vi "pulse data format.vi"(0 "file path (dialog if empty)":path) -> (1 "time":dbl[](array[numeric]) format="%.8f", 2 "file path read":path=path "/Macintosh HD/Data/Jeremy/RbHg/Rb/s12211.001", 3 "rate of change of field":dbl[](array[numeric]) format="%.3f", 4 "magnetic field":dbl[](array[numeric]) format="%.3f", 5 "signal channel A":dbl[](array[numeric]) format="%.3f", 6 "signal channel B":dbl[](array[numeric]) format="%.3f")   [LabVIEW 2016]
uses:
  <vilib>/Analysis/baseanly.llb/Mean (DBL).vi
  <vilib>/Analysis/2dsp.llb/Derivative x(t).vi
  <vilib>/Analysis/NI_AALBase.lvlib
  <vilib>/Analysis/NI_AALPro.lvlib
panel:
  in  "force int?":bool
  in  "B offset":dbl format="%.2f"
  in  "minutes?":bool
  in  "t shift":dbl=0.4 format="%.2f"
  in  "format":string="%f"
  in  "stop":bool
  in  "tau(s)":dbl=0.1 format="%.2f"
  in  "unfilter?":bool
  in  "tau(s)":dbl=0.03 format="%.2f"
  in  "unfilter?":bool
  in  "inv?":bool
  in  "?":u8(ring)=11 items=["1", "3", "7", "15", "31", "63", "127", "255", "511"]
  in  "fit":u16(ring)=2 items=["none", "linear", "box", "auto"]
  in  "sweep rate":dbl=1.0 format="%.2f"
  in  "inv?":bool
  in  "tolerance":dbl=1.0 format="%.2f"
  in  "col":u8=1 min=1
  in  "edit spikes?":bool
  in  "array conversion":u16(ring) items=["standard tab", " arrbitrary spaces"]
  in  "?":i16
  in  "?":i16
  in  "?":bool
  in  "?":bool
  in  "y axis":u16(ring)=3 items=["time", "rate of change of B", "magnetic field", "signal A", "signal B"]
  in  "x axis":u16(ring)=2 items=["time", "rate of change of B", "magnetic field", "signal A", "signal B"]
  out "plotted data":cluster{dbl[], dbl[]}(graph)
  out "no. of columns":u32=5
  out "no. of rows":u32=32768
  in  "y offset":dbl format="%.3f"
  in  "x offset":dbl format="%.3f"
  in  "y col.":u16=3 min=1 step=1
  in  "x col.":u16=2 min=1 step=1
  in  "signal channel B":u16(ring)=3 items=["spreadsheet column x", "integrate column x with constant", "magnitude of columns x & y", "ignore"]
  in  "y offset":dbl format="%.3f"
  in  "x offset":dbl format="%.3f"
  in  "y col.":u16=3 min=1 step=1
  in  "x col.":u16=2 min=1 step=1
  in  "signal channel A":u16(ring) items=["spreadsheet column x", "integrate column x with constant", "magnitude of columns x & y", "Derivative of x column"]
  in  "pretrigger points":u32=1600 min=1 step=1
  in  "column #":u16=2 min=1 step=1
  in  "magnetic field":u16(ring)=2 items=["spreadsheet column", "integrate using time column", " TLM shunt voltage", "field shift correction", "ignore"]
  in  "calibration constant":dbl=11230.0 format="%.2f"
  in  "column #":u16=4 min=1 step=1
  in  "rate of change of field":u16(ring)=1 items=["spreadsheet column", "renormalize column with calibration", "create from B", "ignore"]
  in  "time interval":dbl=2e-06 min=1e-09 format="%.2p"
  in  "column #":u16=5 min=1 step=1
  in  "time column":u16(ring) items=["spreadsheet column", "create from time interval", "ignore"]
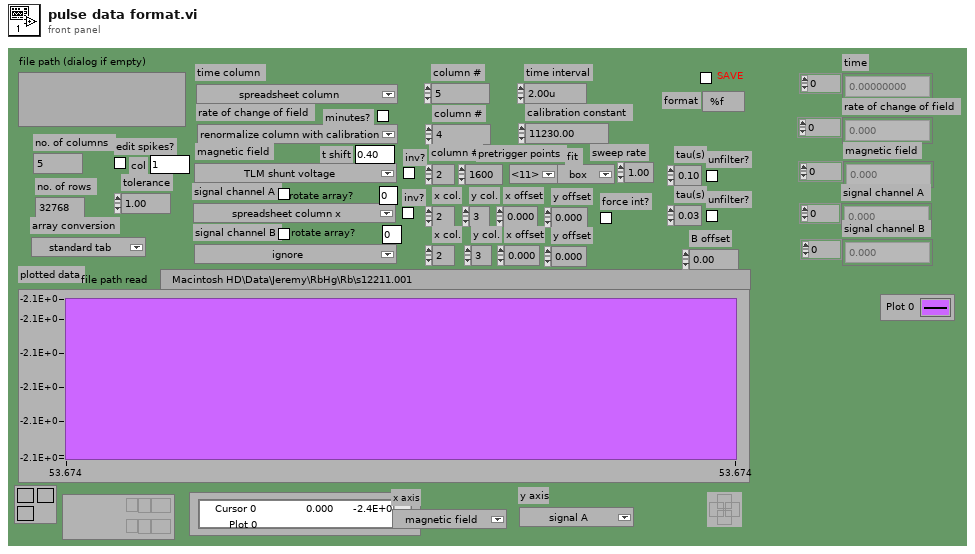
[diagram p1: front panel]
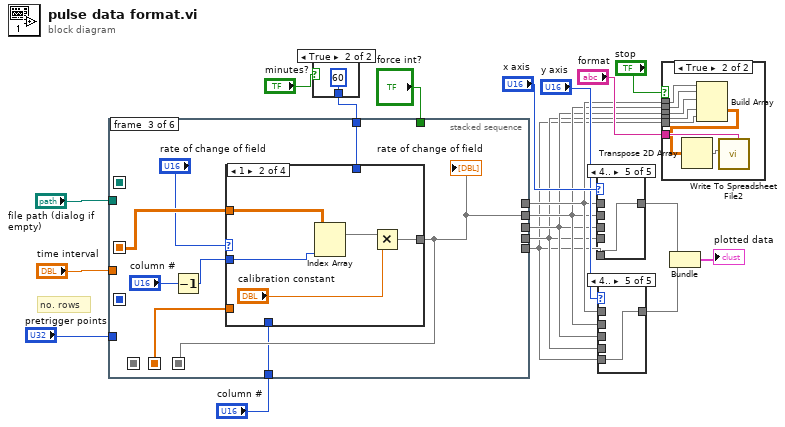
[diagram p0: block diagram]
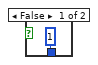
[diagram p2: hidden frame]
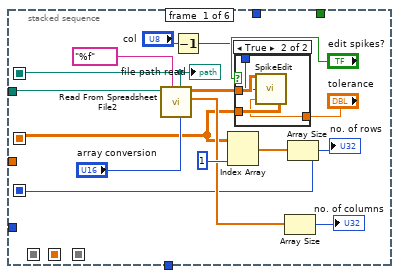
[diagram p12: hidden frame]
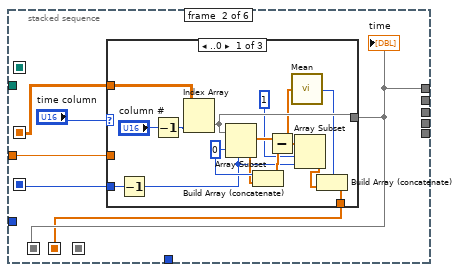
[diagram p14: hidden frame]
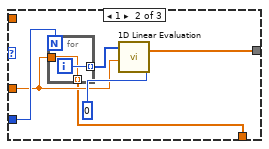
[diagram p15: hidden frame]
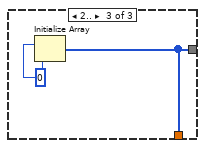
[diagram p16: hidden frame]
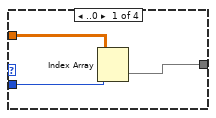
[diagram p17: hidden frame]
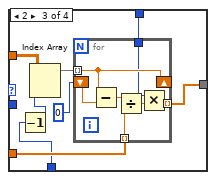
[diagram p18: hidden frame]
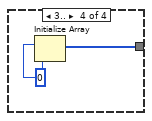
[diagram p19: hidden frame]
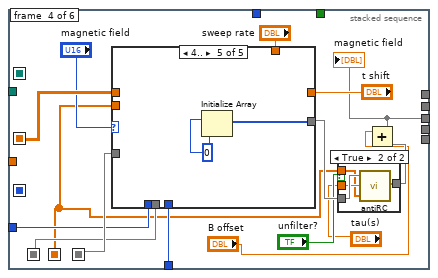
[diagram p20: hidden frame]
diagram:
  # "no. rows"
  n1 = case shown="True" "minutes?" {
    tunnel: [1 60] -> w2
    frame False {
    }
    frame True {
    }
  }
  n2 = stacked-sequence {
    seq-local: [w29 _ _ _ _ _] -> [_ _ _ _ _ _]
    seq-local: [w26 _ _ _ _ _] -> [_ w46 w79 w119 w176 w243]
    seq-local: [w30 _ _ _ _ _] -> [_ w44 _ _ _ _]
    seq-local: [_ w43 _ _ _ _] -> [_ _ _ w117 w162 w232]
    seq-local: [_ _ w75 _ _ _] -> [_ _ _ w118 _ _]
    seq-local: [_ w42 _ _ _ _] -> [_ _ w72 w108 w161 _]
    tunnel: "file path (dialog if empty)" -> [w36 _ _ _ _ _]
    tunnel: "time interval" -> [_ w45 _ _ _ _]
    tunnel: "pretrigger points" -> [_ _ _ w116 w174 w242]
    tunnel: [_ w43 _ _ _ _] -> w9
    tunnel: [_ _ w75 _ _ _] -> w8
    tunnel: [_ _ _ w105 _ _] -> w7
    tunnel: [_ _ _ _ w163 _] -> w6
    tunnel: [_ _ _ _ _ w235] -> w5
    tunnel: "column #" -> [_ _ w74 w109 _ _]
    tunnel: w2 -> [_ _ w73 _ _ _]
    tunnel: "force int?" -> [_ _ _ _ w159 _]
    frame #0 {
      n3 = call "Read From Spreadsheet File2.vi"("array conversion"="array conversion", "format (%.3f)"="%f", "file path (dialog if empty)"=w36) -> ("first row"=w32:sgl[], "all rows"=w27:sgl[][], "new file path (Not A Path if cancelled)"=w29:path)  [unwired: 4 in, 2 out]
      "file path read" <- w29
      n4 = Decrement(x="col") -> (x-1=w23:u8)
      n5 = case shown="True" "edit spikes?" {
        tunnel: w27 -> [w37 w40]
        tunnel: [w37 w41] -> w26
        tunnel: w23 -> [_ w39]
        tunnel: "tolerance" -> [_ w38]
        frame False {
        }
        frame True {
          n6 = call "SpikeEdit.vi"("tolerance"=w38, "column"=w39, "data in"=w40) -> ("data out"=w41:dbl[][])
        }
      }
      n7 = Index Array(array=w26, index (col)=1) -> (element=w33:dbl[])  [unwired: 1 in]
      n8 = Array Size(array=w32) -> (size(s)=→"no. of columns":i32)
      n9 = Array Size(array=w33) -> (size(s)=w30:i32)
      "no. of rows" <- w30
    }
    frame #1 {
      n10 = case shown="..0" "time column" {
        tunnel: [w57 w64 w70] -> w43
        tunnel: w46 -> [w60 _ _]
        tunnel: w45 -> [_ w63 _]
        tunnel: w44 -> [w58 w67 _]
        tunnel: [w48 w62 w70] -> w42
        frame ..0 {
          w56 = 0
          n11 = Decrement(x=w58) -> (x-1=w52:i32)
          n12 = Decrement(x="column #") -> (x-1=w59:u16)
          n13 = Index Array(array=w60, index (col)=w59) -> (element=w57:dbl[])  [unwired: 1 in]
          n14 = Array Subset(array=w57, index=w56, length=w52) -> (w55:dbl[])
          n15 = Build Array (concatenate)(w56, w55) -> (w54:dbl[])
          n16 = Subtract(x=w55, y=w54) -> (x-y=w53:dbl[])
          n17 = call-poly <vilib>:"Mean.vi"("X"=w53) -> ("error"=w50:i32)  [unwired: 1 out]
          n18 = Array Subset(array=w53, index=1, length=w52) -> (w49:dbl[])
          n19 = Build Array (concatenate)(w50, w49) -> (w48:dbl[])
        }
        frame 1 {
          n20 = for {
            N: w67 -> [_]
            tunnel: [w69] -> w66 mode=indexing
            tunnel: w63 -> [w68]
            tunnel: [w68] -> w62 mode=indexing
            i -> [w69]
          }
          n21 = call <vilib>:"1D Linear Evaluation.vi"("offset"=0, "scale"=w63, "X"=w66) -> ("Y[i]=X[i]*a+b"=w64:dbl[])  [unwired: 1 out]
        }
        frame 2.. {
          w71 = 0
          n22 = Initialize Array(w71, w71) -> (w70:i32[])
        }
      }
      "time" <- w43
    }
    frame #2 {
      n23 = Decrement(x="column #") -> (x-1=w76:u16)
      n24 = case shown="1" "rate of change of field" {
        tunnel: [w82 w84 w91 w104] -> w75
        tunnel: w79 -> [w81 w87 w95 _]
        tunnel: w76 -> [w80 w83 _ _]
        tunnel: w72 -> [_ _ w92 _]
        tunnel: w74 -> [_ _ w90 _]
        tunnel: w73 -> [_ _ w88 _]
        frame ..0 {
          n25 = Index Array(array=w81, index (col)=w80) -> (element=w82:dbl[])  [unwired: 1 in]
        }
        frame 1 {
          n26 = Index Array(array=w87, index (col)=w83) -> (element=w85:dbl[])  [unwired: 1 in]
          n27 = Multiply(x=w85, y="calibration constant") -> (x*y=w84:dbl[])
        }
        frame 2 {
          n28 = Decrement(x=w90) -> (x-1=w89:u16)
          n29 = Index Array(array=w95, index (col)=w89) -> (element=w93:dbl[])  [unwired: 1 in]
          n30 = for {
            shift-right: [w102] -> _
            shift-left: 0 -> [w101]
            tunnel: w93 -> [w102] mode=indexing
            tunnel: w92 -> [w99] mode=indexing
            tunnel: [w98] -> w91 mode=indexing
            tunnel: w88 -> [w96]
            n31 = Subtract(x=w102, y=w101) -> (x-y=w100:dbl)
            n32 = Divide(x=w100, y=w99) -> (x/y=w97:dbl)
            n33 = Multiply(x=w96, y=w97) -> (x*y=w98:dbl)
          }
        }
        frame 3.. {
          w103 = 0
          n34 = Initialize Array(w103, w103) -> (w104:i32[])
        }
      }
      "rate of change of field" <- w75
    }
    frame #3 {
      n35 = case shown="4.." "magnetic field" {
        tunnel: [w127 w135 w146 w150 w158] -> w114
        tunnel: w119 -> [w130 _ w149 w154 _]
        tunnel: w116 -> [_ w136 _ _ _]
        tunnel: w118 -> [_ w137 _ _ _]
        tunnel: w108 -> [_ _ _ w151 _]
        tunnel: w117 -> [_ w134 _ _ _]
        tunnel: w109 -> [w126 _ w147 w155 _]
        tunnel: "sweep rate" -> [_ _ w138 _ _]
        tunnel: "t shift" -> [_ _ _ w152 _]
        frame ..0 {
          n36 = Decrement(x=w126) -> (x-1=w129:u16)
          n37 = Index Array(array=w130, index (col)=w129) -> (element=w128:dbl[])  [unwired: 1 in]
          n38 = case shown="True" "inv?" {
            tunnel: w128 -> [w131 w133]
            tunnel: [w131 w132] -> w127
            frame False {
            }
            frame True {
              n39 = Reciprocal(x=w133) -> (1/x=w132:dbl[])
            }
          }
        }
        frame 1 {
          n40 = call "integrator.vi"("pretrigger points"=w136, "time"=w134, "input"=w137) -> ("output"=w135:dbl[])
        }
        frame 2 {
          n41 = Decrement(x=w147) -> (x-1=w148:u16)
          n42 = Index Array(array=w149, index (col)=w148) -> (element=w145:dbl[])  [unwired: 1 in]
          n43 = Increment(x="?") -> (x+1=w142:u8)
          n44 = Scale By Power Of 2(n=w142, x=1) -> (x*2^n=w140:i32)
          n45 = Decrement(x=w140) -> (x-1=w139:i32)
          n46 = call "TLM.vi"("sweep rate (A/min)"=w138, "fit"="fit", "shunt V"=w145, "BOX"=w139) -> ("field (T)"=w146:dbl[])  [unwired: 11 in]
        }
        frame 3 {
          n47 = Decrement(x=w155) -> (x-1=w156:u16)
          n48 = Index Array(array=w154, index (col)=w156) -> (element=w153:dbl[])  [unwired: 1 in]
          n49 = call "fieldshift.vi"("time interval"=w151, "time shift"=w152, "input field"=w153) -> ("outut field"=w150:dbl[])  [unwired: 1 in]
        }
        frame 4.. {
          w157 = 0
          n50 = Initialize Array(w157, w157) -> (w158:i32[])
        }
      }
      n51 = case shown="True" "unfilter?" {
        tunnel: w114 -> [w120 w124]
        tunnel: [w120 w121] -> w107
        tunnel: "tau(s)" -> [_ w123]
        tunnel: w108 -> [_ w122]
        frame False {
        }
        frame True {
          n52 = call "antiRC.vi"("time interval"=w122, "tau"=w123, "in"=w124) -> ("out"=w121:dbl[])
        }
      }
      n53 = Add(x="B offset", y=w107) -> (x+y=w105:dbl[])
      "magnetic field" <- w105
    }
    frame #4 {
      n54 = Decrement(x="x col.") -> (x-1=w173:u16)
      n55 = Decrement(x="y col.") -> (x-1=w171:u16)
      n56 = case shown="1" "signal channel A" {
        tunnel: [w192 w193 w215 w226 w231] -> w169
        tunnel: w176 -> [w191 w208 w223 w228 _]
        tunnel: w173 -> [w190 w207 w224 w229 _]
        tunnel: w162 -> [_ w203 _ _ _]
        tunnel: w174 -> [_ w209 _ _ _]
        tunnel: w171 -> [_ _ w225 _ _]
        tunnel: w159 -> [_ w196 _ _ _]
        frame ..0 {
          n57 = Index Array(array=w191, index (col)=w190) -> (element=w192:dbl[])  [unwired: 1 in]
        }
        frame 1 {
          n58 = Index Array(array=w208, index (col)=w207) -> (element=w206:dbl[])  [unwired: 1 in]
          n59 = Array Size(array=w206) -> (size(s)=w204:i32)
          n60 = Decrement(x=w204) -> (x-1=w201:i32)
          n61 = call "integrator.vi"("pretrigger points"=w209, "time"=w203, "input"=w206) -> ("output"=w194:dbl[])
          n62 = for {
            N: w204 -> [_]
            tunnel: [w214] -> w202 mode=indexing
            i -> [w214]
          }
          n63 = Index Array(array=w194, index=w201) -> (element=w199:dbl)
          n64 = Index Array(array=w194, index=0) -> (element=w200:dbl)
          n65 = Divide(x=w202, y=w201) -> (x/y=w198:dbl[])
          n66 = Subtract(x=w200, y=w199) -> (x-y=w197:dbl)
          n67 = Multiply(x=w198, y=w197) -> (x*y=w195:dbl[])
          n68 = case shown="False" w196 {
            tunnel: w195 -> [_ w213]
            tunnel: w194 -> [w210 w212]
            tunnel: [w210 w211] -> w193
            frame False {
            }
            frame True {
              n69 = Add(x=w213, y=w212) -> (x+y=w211:dbl[])
            }
          }
        }
        frame 2 {
          n70 = Index Array(array=w223, index (col)=w224) -> (element=w222:dbl[])  [unwired: 1 in]
          n71 = Index Array(array=w223, index (col)=w225) -> (element=w221:dbl[])  [unwired: 1 in]
          n72 = Subtract(x=w222, y="x offset") -> (x-y=w218:dbl[])
          n73 = Subtract(x=w221, y="y offset") -> (x-y=w217:dbl[])
          n74 = Re/Im To Complex(1:w217, 2:w218) -> (0:w216:cdb[])
          n75 = Complex To Polar(r * e^(i*theta)=w216) -> (r=w215:dbl[])  [unwired: 1 out]
        }
        frame 3 {
          n76 = Index Array(array=w228, index (col)=w229) -> (element=w227:dbl[])  [unwired: 1 in]
          n77 = call <vilib>:"Derivative x(t) (obs).vi"("X"=w227) -> ("dX/dt"=w226:dbl[])  [unwired: 3 in, 1 out]
        }
        frame 4.. {
          w230 = 0
          n78 = Initialize Array(w230, w230) -> (w231:i32[])
        }
      }
      n79 = case shown="True" "?" {
        tunnel: [w186 w187] -> w166
        tunnel: w169 -> [w186 w189]
        tunnel: "?" -> [_ w188]
        frame False {
        }
        frame True {
          n80 = Rotate 1D Array(1:w189, 2:w188) -> (0:w187:dbl[])
        }
      }
      n81 = case shown="True" "inv?" {
        tunnel: [w183 w184] -> w164
        tunnel: w166 -> [w183 w185]
        frame False {
        }
        frame True {
          n82 = Negate(x=w185) -> (-x=w184:dbl[])
        }
      }
      n83 = case shown="True" "unfilter?" {
        tunnel: w164 -> [w178 w182]
        tunnel: [w178 w179] -> w163
        tunnel: "tau(s)" -> [_ w181]
        tunnel: w161 -> [_ w180]
        frame False {
        }
        frame True {
          n84 = call "antiRC.vi"("time interval"=w180, "tau"=w181, "in"=w182) -> ("out"=w179:dbl[])
        }
      }
      "signal channel A" <- w163
    }
    frame #5 {
      n85 = Decrement(x="y col.") -> (x-1=w240:u16)
      n86 = Decrement(x="x col.") -> (x-1=w241:u16)
      n87 = case shown="1" "signal channel B" {
        tunnel: [w250 w256 w259 w269] -> w236
        tunnel: w243 -> [w249 w253 w265 _]
        tunnel: w241 -> [w248 w252 w266 _]
        tunnel: w232 -> [_ w255 _ _]
        tunnel: w242 -> [_ w254 _ _]
        tunnel: w240 -> [_ _ w267 _]
        frame ..0 {
          n88 = Index Array(array=w249, index (col)=w248) -> (element=w250:dbl[])  [unwired: 1 in]
        }
        frame 1 {
          n89 = Index Array(array=w253, index (col)=w252) -> (element=w251:dbl[])  [unwired: 1 in]
          n90 = call "integrator.vi"("pretrigger points"=w254, "time"=w255, "input"=w251) -> ("output"=w256:dbl[])
        }
        frame 2 {
          n91 = Index Array(array=w265, index (col)=w266) -> (element=w264:dbl[])  [unwired: 1 in]
          n92 = Index Array(array=w265, index (col)=w267) -> (element=w263:dbl[])  [unwired: 1 in]
          n93 = Subtract(x=w264, y="x offset") -> (x-y=w262:dbl[])
          n94 = Subtract(x=w263, y="y offset") -> (x-y=w261:dbl[])
          n95 = Re/Im To Complex(1:w261, 2:w262) -> (0:w260:cdb[])
          n96 = Complex To Polar(r * e^(i*theta)=w260) -> (r=w259:dbl[])  [unwired: 1 out]
        }
        frame 3.. {
          w268 = 0
          n97 = Initialize Array(w268, w268) -> (w269:i32[])
        }
      }
      n98 = case shown="True" "?" {
        tunnel: [w244 w245] -> w235
        tunnel: w236 -> [w244 w247]
        tunnel: "?" -> [_ w246]
        frame False {
        }
        frame True {
          n99 = Rotate 1D Array(1:w247, 2:w246) -> (0:w245:dbl[])
        }
      }
      "signal channel B" <- w235
    }
  }
  n100 = case shown="4.." "x axis" {
    tunnel: w9 -> [w270 _ _ _ _]
    tunnel: w8 -> [_ w271 _ _ _]
    tunnel: w7 -> [_ _ w272 _ _]
    tunnel: w6 -> [_ _ _ w273 _]
    tunnel: w5 -> [_ _ _ _ w274]
    tunnel: [w270 w271 w272 w273 w274] -> w13
    frame ..0 {
    }
    frame 1 {
    }
    frame 2 {
    }
    frame 3 {
    }
    frame 4.. {
    }
  }
  n101 = case shown="4.." "y axis" {
    tunnel: w9 -> [w275 _ _ _ _]
    tunnel: w8 -> [_ w276 _ _ _]
    tunnel: w7 -> [_ _ w277 _ _]
    tunnel: w6 -> [_ _ _ w278 _]
    tunnel: w5 -> [_ _ _ _ w279]
    tunnel: [w275 w276 w277 w278 w279] -> w12
    frame ..0 {
    }
    frame 1 {
    }
    frame 2 {
    }
    frame 3 {
    }
    frame 4.. {
    }
  }
  n102 = case shown="True" "stop" {
    tunnel: "format" -> [_ w286]
    tunnel: w9 -> [_ w285]
    tunnel: w8 -> [_ w284]
    tunnel: w7 -> [_ w283]
    tunnel: w6 -> [_ w282]
    tunnel: w5 -> [_ w281]
    frame False {
    }
    frame True {
      n103 = Build Array(w285, w284, w283, w282, w281) -> (w280:dbl[][])
      n104 = Transpose 2D Array(2D array=w280) -> (transposed array=w287:dbl[][])
      n105 = call "Write To Spreadsheet File2.vi"("format (%.3f)"=w286, "2D data"=w287) -> ()  [unwired: 6 in, 1 out]
    }
  }
  n106 = Bundle("output"=w13, "output"=w12) -> (→"plotted data":cluster{"output":dbl[], "output":dbl[]})  [unwired: 1 in]
